vi "Add Tx Queue Status Section.vi"(8 "error in":errorcluster, 11 "Section Ref in":T1 format="%.0x") -> (0 "error out":errorcluster, 1 "Tx Queue Status channel Refs":T1[](array[typedef]) format="%.0x", 2 "Tx Queue Status Section Ref out":T1 format="%.0x", 3 "Section Ref out":T1 format="%.0x")   [LabVIEW 2020, in "AIM ARINC 664 Scripting.lvlib"]
uses:
  AIM ARINC 664 Scripting.lvlib
  <vilib>/NI VeriStand/Custom Device API/Custom Device Item Ref.ctl
  <vilib>/NI VeriStand/Custom Device API/Custom Device Channel.ctl
  <vilib>/NI VeriStand/Custom Device API/Custom Device Channel Type.ctl
  Controls/Tx Generic Queue Status Enum.ctl
  Constants.vi
  <vilib>/NI VeriStand/Custom Device API/Custom Device API.lvlib
  <vilib>/NI/NI VeriStand Advanced SysDef API/SysDef API/Advanced System Definition.lvlib
  <vilib>/Utility/Data Type/NI_Data Type.lvlib
  GUID Utility/AIM ARINC 664 GUID Utility.lvlib
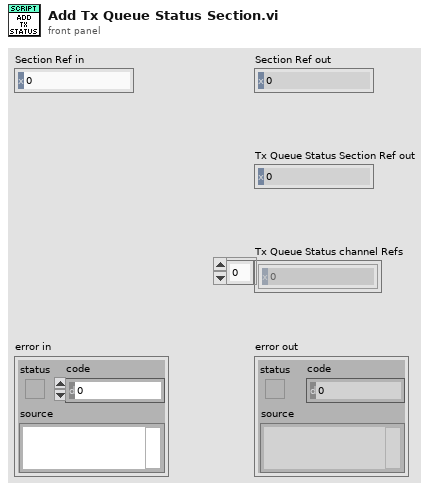
[diagram p1: front panel]
types:
  T1 = typedef "Custom Device API.lvlib/Custom Device Item Ref.ctl" = u64
  T2 = typedef "Tx Generic Queue Status Enum.ctl" = enum16{"FDX_QUE_EMPTY", "FDX_QUE_FILLED", "FDX_QUE_FULL", "FDX_QUE_SENT", "FDX_QUE_CYCL_RUN", "FDX_QUE_CYCL_SENT"}
  T3 = typedef "Custom Device API.lvlib/Custom Device Channel.ctl" = cluster{"Type":T4, "Units":string, "Default Value":dbl, "Faultable":bool, "Scalable":bool}
  T4 = typedef "Custom Device API.lvlib/Custom Device Channel Type.ctl" = enum16{"Input", "Output"}
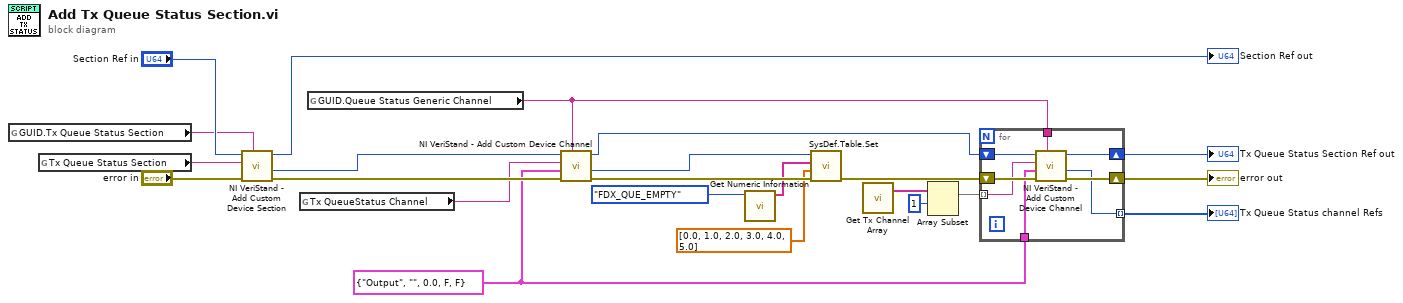
[diagram p0: block diagram]
diagram:
  w10 = T3 {"Type"=enum."Output", "Units"="", "Default Value"=0.0, "Faultable"=FALSE, "Scalable"=FALSE} ("Channel")
  n1 = global read "Constants.vi" "GUID.Tx Queue Status Section"() -> (w19:string)
  n2 = global read "Constants.vi" "Tx Queue Status Section"() -> (w21:string)
  n3 = call <vilib>:"NI VeriStand - Add Custom Device Section.vi"("GUID (Default Section)"=w19, "error in (no error)"="error in", "Section Name"=w21, "Parent Ref in"="Section Ref in") -> ("error out"=w20:errorcluster, "Section Ptr"=w14:T1, "Parent Ref out"=→"Section Ref out":T1)  [unwired: 4 in, 1 out]
  n4 = global read "Constants.vi" "Tx QueueStatus Channel"() -> (w11:string)
  n5 = global read "Constants.vi" "GUID.Queue Status Generic Channel"() -> (w12:string)
  n6 = call <vilib>:"NI VeriStand - Add Custom Device Channel.vi"("GUID (Default Channel)"=w12, "error in (no error)"=w20, "Channel"=w10, "Channel Name"=w11, "Parent Ref in"=w14) -> ("error out"=w9:errorcluster, "Channel Ref"=w7:T1, "Parent Ref out"=w13:T1)  [unwired: 3 in, 1 out]
  n7 = call <vilib>:"Get Numeric Information.vi"("variant"=Tx_Generic_Queue_Status_Enum."FDX_QUE_EMPTY") -> ("enum names"=w6:string[])  [unwired: 7 in, 3 out]
  n8 = call <vilib>:"SysDef.Table.Set.vi"("error in (no error)"=w9, "Values"=dbl[] [0.0, 1.0, 2.0, 3.0, 4.0, 5.0], "Names"=w6, "nodeID"=w7) -> ("error out"=w8:errorcluster)  [unwired: 6 in, 1 out]
  n9 = call "Get Tx Channel Array.vi"() -> ("Channel Array"=w3:string[])  [unwired: 3 in]
  n10 = Array Subset(array=w3, index=1) -> (w2:string[])  [unwired: 1 in]
  n11 = for {
    tunnel: [w27] -> w15 mode=indexing
    shift-right: [w28] -> w16
    shift-left: w8 -> [w31]
    tunnel: w2 -> [w26] mode=indexing
    tunnel: w10 -> [w25]
    tunnel: w12 -> [w24]
    shift-right: [w30] -> w18
    shift-left: w13 -> [w29]
    n12 = call <vilib>:"NI VeriStand - Add Custom Device Channel.vi"("GUID (Default Channel)"=w24, "error in (no error)"=w31, "Channel"=w25, "Channel Name"=w26, "Parent Ref in"=w29) -> ("error out"=w28:errorcluster, "Channel Ref"=w27:T1, "Parent Ref out"=w30:T1)  [unwired: 3 in, 1 out]
  }
  "Tx Queue Status Section Ref out" <- w18
  "error out" <- w16
  "Tx Queue Status channel Refs" <- w15
